vi "access数据转JOSN发送.vi"() -> ()   [LabVIEW 2016]
uses:
  <vilib>/httpClient/POSTBuffer.vi
  <vilib>/Utility/config.llb/NI_LVConfig.lvlib
  <vilib>/httpClient/LabVIEWHTTPClient.lvlib
  <vilib>/ptbypt/NI_PtbyPt.lvlib
panel:
  in  "数据补传":bool
  out "元素":string
  out "date/time string":string
  out "队列中元素数量":i32
  in  "开机启动":bool
  out "body":string caption="体部"
  out "headers":string caption="头部"
  in  "url":string="127.0.0.1:1000"
  out "error out":errorcluster
  in  "station_id":string="AH CODCR"
  in  "time":string="2021-05-08 14:02:02"
  in  "查询":bool
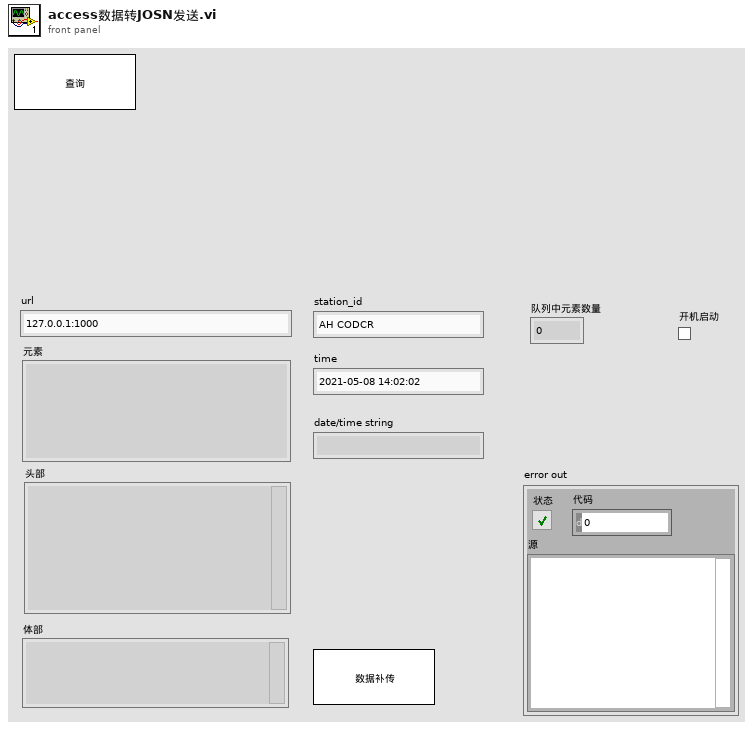
[diagram p1: front panel]
types:
  T1 = typedef "LVDateTimeRec.ctl" = cluster{"秒数的小数部分":dbl, "秒":i32, "分":i32, "时":i32, "日":i32, "月":i32, "年":i32, "天数（周）":i32, "天数（年）":i32, "DST":i32}
  T2 = typedef "NI_LVConfig.lvlib/Config Data RefNum.ctl" = refnum<k1>
  T3 = cluster{"CODCr":string[][], "氨氮":string[][], "总磷":string[][], "总氮":string[][], "CODMn":string[][], "DO":string[][], "PH":string[][], "水温":string[][], "浊度":string[][], "电导率":string[][], "氟化物":string[][]}
  T4 = typedef "LabVIEWHTTPClient.lvlib/ClientHandle.ctl" = refnum<k1>
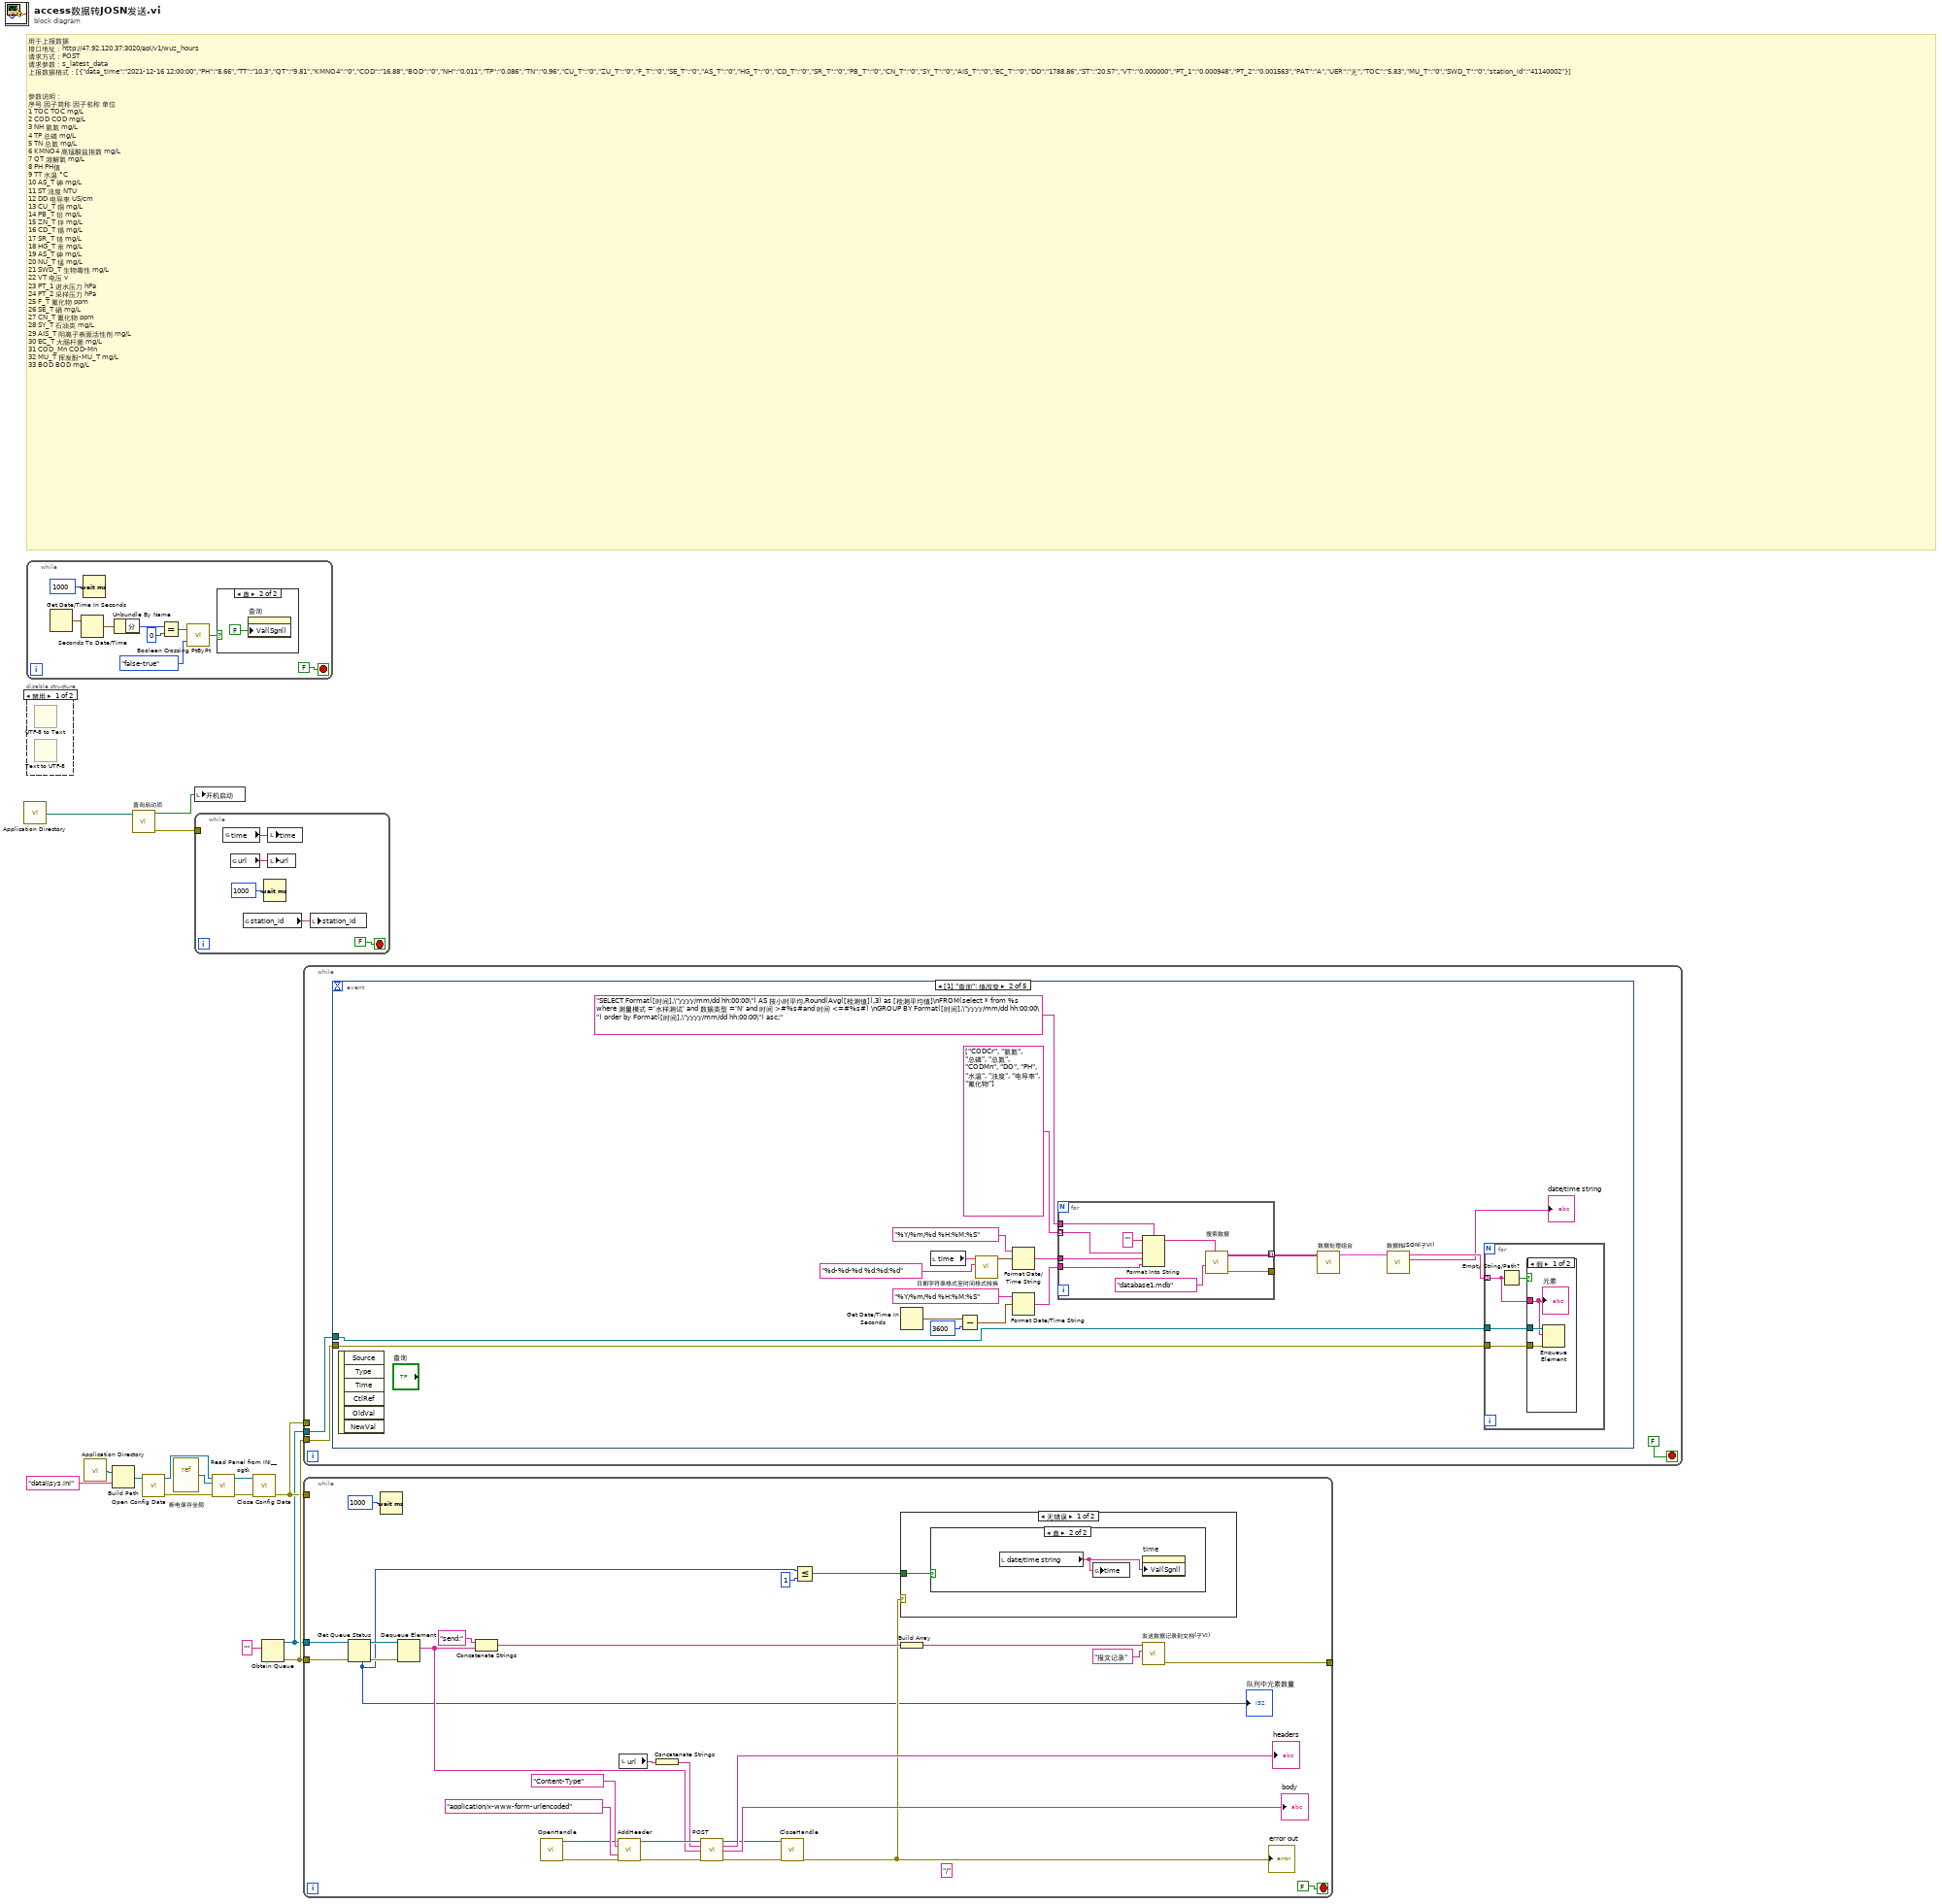
[diagram p0: block diagram]
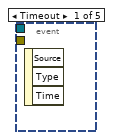
[diagram p6: hidden frame]
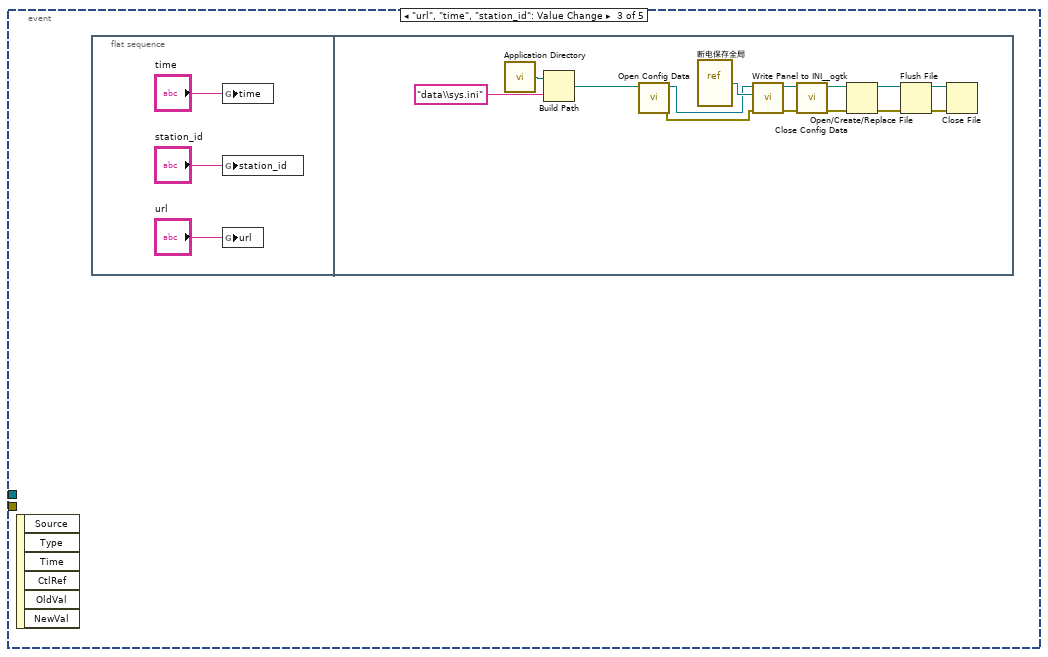
[diagram p8: hidden frame]
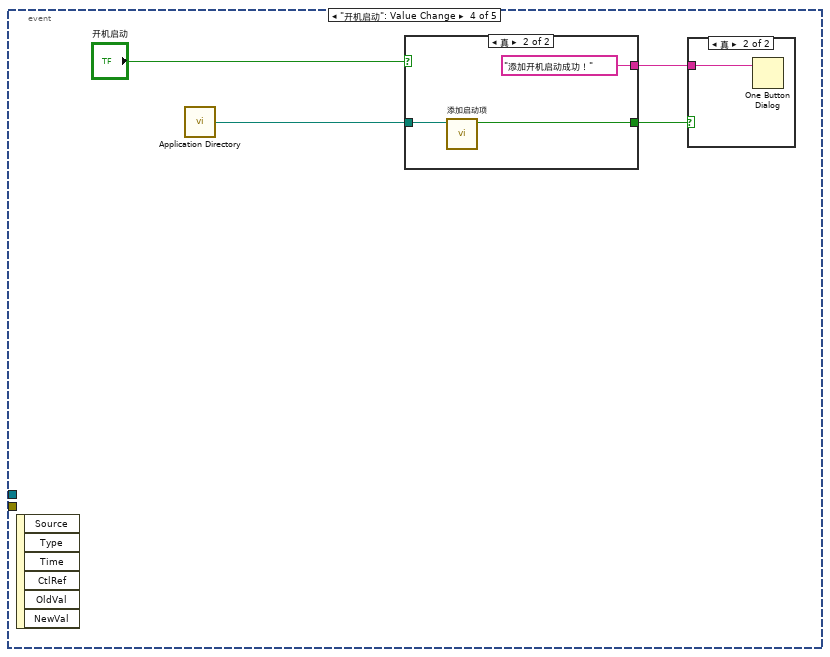
[diagram p9: hidden frame]
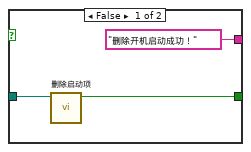
[diagram p11: hidden frame]
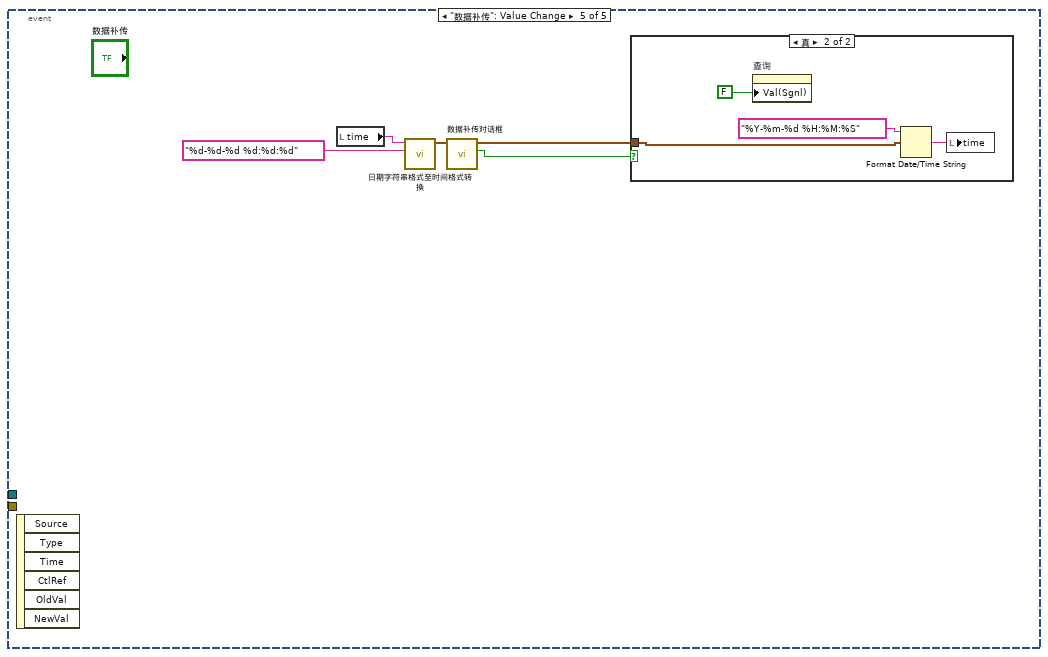
[diagram p12: hidden frame]
diagram:
  # "用于上报数据 \n接口地址：http://47.92.120.37:3020/api/v1/wuz_hours\n请求方式：POST \n请求参数：s_latest_data\n上报数据格式：[{\"data_time\":\"2021-12-16 12:00:00\",\"PH\":\"8.66\",\"TT\":\"10.3\",\"QT\":\"9.81\",\"KMNO4\":\"0\",\"COD\":\"16.88\",\"BOD\":\"0\",\"NH\":\"0.011\",\"TP\":\"0.086\",\"TN\":\"0.96\",\"CU_T\":\"0\",\"ZU_T\":\"0\",\"F_T\":\"0\",\"SE_T\":\"0\",\"AS_T\":\"0\",\"HG_T\":\"0\",\"CD_T\":\"0\",\"SR_T\":\"0\",\"PB_T\":\"0\",\"CN_T\":\"0\",\"SY_T\":\"0\",\"AIS_T\":\"0\",\"EC_T\":\"0\",\"DD\":\"1788.86\",\"ST\":\"20.57\",\"VT\":\"0.000000\",\"PT_1\":\"0.000948\",\"PT_2\":\"0.001563\",\"PAT\":\"A\",\"UER\":\"无\",\"TOC\":\"5.83\",\"MU_T\":\"0\",\"SWD_T\":\"0\",\"station_id\":\"41140002\"}]\n\n\n参数说明：\n序号\t因子简称\t因子名称\t单位\n1\tTOC\tTOC\tmg/L\n2\tCOD\tCOD\tmg/L\n3\tNH\t氨氮\tmg/L\n4\tTP\t总磷\tmg/L\n5\tTN\t总氮\tmg/L\n6\tKMNO4\t高锰酸盐指数\tmg/L\n7\tQT\t溶解氧\tmg/L\n8\tPH\tPH值\t\n9\tTT\t水温\t°C\n10\tAS_T\t砷\tmg/L\n11\tST\t浊度\tNTU\n12\tDD\t电导率\tUS/cm\n13\tCU_T\t铜\tmg/L\n14\tPB_T\t铅\tmg/L\n15\tZN_T\t锌\tmg/L\n16\tCD_T\t镉\tmg/L\n17\tSR_T\t铬\tmg/L\n18\tHG_T\t汞\tmg/L\n19\tAS_T\t砷\tmg/L\n20\tNU_T\t锰\tmg/L\n21\tSWD_T\t生物毒性\tmg/L\n22\tVT\t电压\tv\n23\tPT_1\t进水压力\thPa\n24\tPT_2\t采样压力\thPa\n25\tF_T\t氟化物\tppm\n26\tSE_T\t硒\tmg/L\n27\tCN_T\t氰化物\tppm\n28\tSY_T\t石油类\tmg/L\n29\tAIS_T\t阴离子表面活性剂\tmg/L\n30\tEC_T\t大肠杆菌\tmg/L\n31\tCOD_Mn\tCOD-Mn\t\n32\tMU_T\t挥发酚-MU_T\tmg/L\n33\tBOD\tBOD\tmg/L"
  n1 = call <vilib>:"Application Directory.vi"() -> ("Application Directory"=w3:path)
  n2 = while {
    stop <- FALSE stop-if-true
    n3 = Get Date/Time In Seconds() -> (seconds since 1Jan1904=w21:timestamp)
    n4 = Seconds To Date/Time(time stamp (now)=w21) -> (date time rec=w22:T1)  [unwired: 1 in]
    n5 = Wait (ms)(milliseconds to wait=u32 1000 ("等待时间（毫秒）")) -> ()  [unwired: 1 out]
    n6 = Unbundle By Name(w22) -> ("分"=w20:i32)
    n7 = Equal?(x=w20, y=0) -> (x = y?=w18:bool)
    n8 = call <vilib>:"Boolean Crossing PtByPt.vi"("direction"=enum16{"either", "false-true", "true-false"}."false-true", "input"=w18) -> ("crossing"=w16:bool)  [unwired: 1 in]
    n9 = case shown="真" w16 {
      frame False {
      }
      frame True {
        n10 = property on="查询" class="Bool (严格)"("Val(Sgnl)"=FALSE ("值(信号)")) -> ()  [unwired: 2 in, 2 out]
      }
    }
  }
  n11 = disable-structure shown="禁用" {
    frame Disabled {
      n12 = UTF-8 to Text() -> ()  [unwired: 3 in, 2 out]
      n13 = Text to UTF-8() -> ()  [unwired: 3 in, 2 out]
    }
    frame Enabled {
    }
  }
  n14 = call <vilib>:"Application Directory.vi"() -> ("Application Directory"=w10:path)
  n15 = Build Path(base path=w10, name or relative path="data\\sys.ini" ("名称或相对路径")) -> (appended path=w9:path)
  n16 = call "查询启动项.vi"("启动文件路径"=w3) -> ("error out"=w2:errorcluster, "包含启动项"=w4:bool)  [unwired: 9 in]
  n17 = call <vilib>:"Open Config Data.vi"("configuration file path"=w9) -> ("error out"=w13:errorcluster, "refnum"=w12:T2)  [unwired: 8 in, 1 out]
  n18 = vi-ref "断电保存全局.vi"() -> (w7:refnum<vi>)
  n19 = local write "开机启动"(w4) -> ()
  n20 = while {
    tunnel: w2 -> [_]
    stop <- FALSE stop-if-true
    n21 = global read "断电保存全局.vi" "time"() -> (w27:string)
    n22 = global read "断电保存全局.vi" "url"() -> (w28:string)
    n23 = global read "断电保存全局.vi" "station_id"() -> (w26:string)
    n24 = Wait (ms)(milliseconds to wait=u32 1000 ("等待时间（毫秒）")) -> ()  [unwired: 1 out]
    n25 = local write "time"(w27) -> ()
    n26 = local write "url"(w28) -> ()
    n27 = local write "station_id"(w26) -> ()
  }
  n28 = call <userlib>:"Read Panel from INI__ogtk.vi"("error in (no error)"=w13, "VI ref"=w7, "refnum"=w12) -> ("error out"=w8:errorcluster, "refnum out"=w11:T2)  [unwired: 7 in]
  n29 = call <vilib>:"Close Config Data.vi"("error in (no error)"=w8, "refnum"=w11) -> ("error out"=w5:errorcluster)  [unwired: 8 in, 1 out]
  n30 = Obtain Queue(element data type="") -> (queue out=w1:refnum<queue>, error out=w15:errorcluster)  [unwired: 4 in, 1 out]
  n31 = while {
    tunnel: w1 -> [w33]
    tunnel: w15 -> [w32]
    tunnel: w5 -> [_]
    stop <- FALSE stop-if-true
    n32 = event shown="[1] \"查询\": 值改变" {
      selector: _ -> [_ _ _ _ _]
      dyn-events: _ -> [_ _ _ _ _]
      timeout: _ -> [_ _ _ _ _]
      tunnel: w33 -> [_ w36 _ _ _]
      tunnel: w32 -> [_ w35 _ _ _]
      event Timeout {
        n33 = event-data() -> ()  [unwired: 1 in, 3 out]
      }
      event "查询": Value Change {
        n34 = event-data() -> ()  [unwired: 1 in, 6 out]
        n35 = Get Date/Time In Seconds() -> (seconds since 1Jan1904=w46:timestamp)
        n36 = local read "time"() -> (w50:string)
        n37 = Subtract(x=w46, y=3600) -> (x-y=w44:timestamp)
        n38 = call "日期字符串格式至时间格式转换.vi"("格式字符串"="%d-%d-%d %d:%d:%d", "time"=w50) -> ("time stamp"=w47:timestamp)  [unwired: 9 in]
        n39 = Format Date/Time String(time format string (%c)="%Y/%m/%d %H:%M:%S" ("时间格式字符串(%c)"), seconds (now)=w47) -> (date/time string=w41:string)  [unwired: 1 in]
        n40 = Format Date/Time String(time format string (%c)="%Y/%m/%d %H:%M:%S" ("时间格式字符串(%c)"), seconds (now)=w44) -> (date/time string=w40:string)  [unwired: 1 in]
        n41 = for {
          tunnel: string[] ["CODCr", "氨氮", "总磷", "总氮", "CODMn", "DO", "PH", "水温", "浊度", "电导率", "氟化物"] -> [w63] mode=indexing
          tunnel: "SELECT Format([时间],\"yyyy/mm/dd hh:00:00\") AS 按小时平均,Round(Avg([检测值]),3) as [检测平均值]\nFROM(select * from %s where 测量模式 ='水样测试' and 数据类型 ='N' and 时间 >#%s#and 时间 <=#%s#) \nGROUP BY Format([时间],\"yyyy/mm/dd hh:00:00\") order by Format([时间],\"yyyy/mm/dd hh:00:00\") asc;" ("condition") -> [w66]
          tunnel: w41 -> [w65]
          tunnel: w40 -> [w64]
          tunnel: [w60] -> w39 mode=indexing
          tunnel: [w59] -> _
          n42 = Format Into String(format string=w66, initial string="" ("初始字符串"), w63, w65, w64) -> (resulting string=w62:string)  [unwired: 1 in, 1 out]
          n43 = call "搜索数据.vi"("condition"=w62, "database"="database1.mdb") -> ("error out"=w59:errorcluster, "data"=w60:string[][])  [unwired: 8 in]
        }
        n44 = call "数据处理组合.vi"("待排序数组"=w39) -> ("输出簇"=w38:T3)  [unwired: 10 in]
        n45 = call "数据转JSON(子VI).vi"("输出簇"=w38) -> ("result string"=→"date/time string":string, "数组"=w37:string[])  [unwired: 9 in]
        n46 = for {
          tunnel: w37 -> [w53] mode=indexing
          tunnel: w36 -> [w54]
          tunnel: w35 -> [w52]
          n47 = Empty String/Path?(string/path=w53) -> (empty?=w55:bool)
          n48 = case shown="假" w55 {
            tunnel: w54 -> [w58 _]
            tunnel: w53 -> [w56 _]
            tunnel: w52 -> [w57 _]
            frame False {
              n49 = Enqueue Element(queue=w58, element=w56, error in (no error)=w57) -> ()  [unwired: 1 in, 3 out]
              "元素" <- w56
            }
            frame True {
            }
          }
        }
      }
      event "url", "time", "station_id": Value Change {
        n50 = event-data() -> ()  [unwired: 1 in, 6 out]
        n51 = flat-sequence {
          frame #0 {
            n52 = global write "断电保存全局.vi" "time"("time") -> ()
            n53 = global write "断电保存全局.vi" "station_id"("station_id") -> ()
            n54 = global write "断电保存全局.vi" "url"("url") -> ()
          }
          frame #1 {
            n55 = call <vilib>:"Application Directory.vi"() -> ("Application Directory"=w71:path)
            n56 = Build Path(base path=w71, name or relative path="data\\sys.ini" ("名称或相对路径")) -> (appended path=w73:path)
            n57 = call <vilib>:"Open Config Data.vi"("configuration file path"=w73) -> ("error out"=w77:errorcluster, "refnum"=w74:T2)  [unwired: 8 in, 1 out]
            n58 = vi-ref "断电保存全局.vi"() -> (w75:refnum<vi>)
            n59 = call <userlib>:"Write Panel to INI__ogtk.vi"("error in (no error)"=w77, "VI ref"=w75, "refnum"=w74) -> ("error out"=w78:errorcluster, "refnum out"=w76:T2)  [unwired: 7 in]
            n60 = call <vilib>:"Close Config Data.vi"("error in (no error)"=w78, "refnum"=w76) -> ("error out"=w83:errorcluster, "file path"=w84:path)  [unwired: 8 in]
            n61 = Open/Create/Replace File(file path (use dialog)=w84, error in=w83) -> (refnum out=w80:refnum<file>, error out=w79:errorcluster)  [unwired: 4 in, 1 out]
            n62 = Flush File(refnum=w80, error in=w79) -> (refnum out=w81:refnum<file>, error out=w82:errorcluster)
            n63 = Close File(refnum=w81, error in=w82) -> ()  [unwired: 2 out]
          }
        }
      }
      event "开机启动": Value Change {
        n64 = event-data() -> ()  [unwired: 1 in, 6 out]
        n65 = call <vilib>:"Application Directory.vi"() -> ("Application Directory"=w87:path)
        n66 = case shown="真" "开机启动" {
          tunnel: w87 -> [w92 w95]
          tunnel: [w91 w94] -> w86
          tunnel: ["删除开机启动成功！" ("消息") "添加开机启动成功！" ("消息")] -> w85
          frame False {
            n67 = call "删除启动项.vi"("启动文件路径"=w92) -> ("删除标记"=w91:bool)  [unwired: 9 in, 1 out]
          }
          frame True {
            n68 = call "添加启动项.vi"("启动文件路径"=w95) -> ("添加成功标记"=w94:bool)  [unwired: 9 in, 1 out]
          }
        }
        n69 = case shown="真" w86 {
          tunnel: w85 -> [_ w89]
          frame False {
          }
          frame True {
            n70 = One Button Dialog(message=w89) -> ()  [unwired: 1 in, 1 out]
          }
        }
      }
      event "数据补传": Value Change {
        n71 = event-data() -> ()  [unwired: 1 in, 6 out]
        n72 = local read "time"() -> (w99:string)
        n73 = call "日期字符串格式至时间格式转换.vi"("格式字符串"="%d-%d-%d %d:%d:%d", "time"=w99) -> ("time stamp"=w98:timestamp)  [unwired: 9 in]
        n74 = call "数据补传对话框.vi"("数据发送时间"=w98) -> ("布尔"=w97:bool, "数据发送时间输出"=w96:timestamp)  [unwired: 9 in]
        n75 = case shown="真" w97 {
          tunnel: w96 -> [_ w103]
          frame False {
          }
          frame True {
            n76 = property on="查询" class="Bool (严格)"("Val(Sgnl)"=FALSE ("值(信号)")) -> ()  [unwired: 2 in, 2 out]
            n77 = Format Date/Time String(time format string (%c)="%Y-%m-%d %H:%M:%S" ("时间格式字符串(%c)"), seconds (now)=w103) -> (date/time string=w102:string)  [unwired: 1 in]
            n78 = local write "time"(w102) -> ()
          }
        }
      }
    }
  }
  n79 = while {
    tunnel: w1 -> [w111]
    tunnel: w15 -> [w110]
    tunnel: w5 -> [_]
    tunnel: [w125] -> _
    stop <- FALSE stop-if-true
    (unwired) "/" ("字符串")
    n80 = Get Queue Status(queue=w111, error in (no error)=w110) -> (queue out=w109:refnum<queue>, error out=w108:errorcluster, # elements in queue=w107:i32)  [unwired: 1 in, 5 out]
    "队列中元素数量" <- w107
    n81 = Wait (ms)(milliseconds to wait=u32 1000 ("等待时间（毫秒）")) -> ()  [unwired: 1 out]
    n82 = Dequeue Element(queue=w109, error in (no error)=w108) -> (element=w113:string)  [unwired: 1 in, 3 out]
    n83 = Concatenate Strings("send:" ("字符串"), w113) -> (w128:string)
    n84 = call <vilib>:"OpenHandle.vi"() -> ("client handle out"=w120:T4, "error out"=w119:errorcluster)  [unwired: 14 in]
    n85 = call <vilib>:"AddHeader.vi"("client handle"=w120, "header"="Content-Type", "value"="application/x-www-form-urlencoded", "error in (no error)"=w119) -> ("client handle out"=w121:T4, "error out"=w122:errorcluster)  [unwired: 10 in]
    n86 = local read "url"() -> (w114:string)
    n87 = Concatenate Strings(w114) -> (w115:string)
    n88 = call-poly <vilib>:"POST.vi"("client handle"=w121, "url"=w115, "buffer"=w113, "error in (no error)"=w122) -> ("client handle out"=w118:T4, "headers"=→"headers":string, "body"=→"body":string, "error out"=w117:errorcluster)  [unwired: 8 in]
    n89 = call <vilib>:"CloseHandle.vi"("client handle"=w118, "error in (no error)"=w117) -> ("error out"=w116:errorcluster)  [unwired: 13 in]
    "error out" <- w116
    n90 = Less Or Equal?(x=w107, y=1) -> (x <= y?=w105:bool)
    n91 = case shown="无错误" w116 {
      tunnel: w105 -> [w133 _]
      frame No Error {
        n92 = case shown="真" w133 {
          frame False {
          }
          frame True {
            n93 = local read "date/time string"() -> (w134:string)
            n94 = global write "断电保存全局.vi" "time"(w134) -> ()
            n95 = property on="time" class="Str"("Val(Sgnl)"=w134) -> ()  [unwired: 2 in, 2 out]
          }
        }
      }
      frame Error {
      }
    }
    n96 = Build Array(w128) -> (w127:string[])
    n97 = call "发送数据记录到文档(子VI).vi"("字符串"="报文记录", "数组"=w127) -> ("错误输出"=w125:errorcluster)  [unwired: 8 in]
  }
